vi "Array To Matrix - RA.vi"(1 "Real 1D Array":dbl[](array[numeric])) -> (0 "Real Matrix (Column Vector)":T1)   [LabVIEW 2017, in "NI_Matrix.lvlib"]
doc: "Converts an array to a matrix of elements of the same type as the array elements. Wire data to the <B>Real 2D Array</B> input to determine the polymorphic instance to use or manually select the instance."
uses:
  NI_Matrix.lvlib
  RealMatrix.ctl
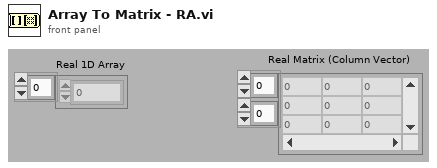
[diagram p1: front panel]
types:
  T1 = typedef "NI_Matrix.lvlib/RealMatrix.ctl" = dbl[][]
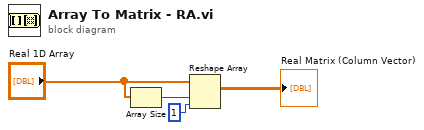
[diagram p0: block diagram]
diagram:
  n1 = Array Size(array="Real 1D Array") -> (size(s)=w4:i32)
  n2 = Reshape Array("Real 1D Array", w4, 1 ("dimension size")) -> (→"Real Matrix (Column Vector)":dbl[][])
